vi "Configure Function Mode of Source.vi"(8 "error in":errorcluster, 10 "Mode":u16(ring) items=["Fixed", "List", "Battery", "Solar", "CarProfile", "Fuel", "Step"], 11 "VISA resource name":refnum<visa-resource-name>) -> (0 "error out":errorcluster, 3 "VISA resource name out":refnum<visa-resource-name>)   [LabVIEW 2015, in "IT-M3900C.lvlib"]
doc: "This command is used to set the power supply function mode.\n<b>Mode</b>\n0:Fixed\n1:List\n2:Battery\n3:Solar\n4:CarProfile\n5:Fuel\n6:Step"
uses:
  <instrlib>/IT-M3900C/IT-M3900C.lvlib
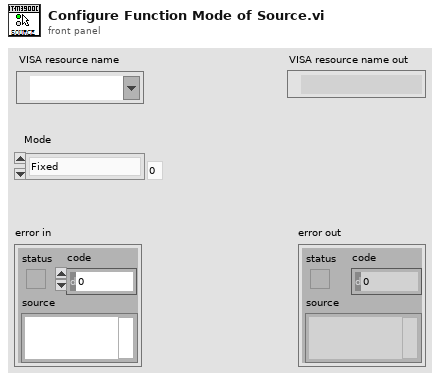
[diagram p1: front panel]
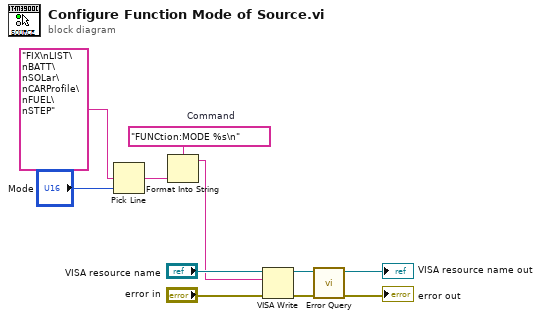
[diagram p0: block diagram]
diagram:
  w5 = "FUNCtion:MODE %s\n"  # Command
  n1 = Pick Line(multi-line string="FIX\nLIST\nBATT\nSOLar\nCARProfile\nFUEL\nSTEP", line index="Mode") -> (output string=w1:string)  [unwired: 1 in]
  n2 = Format Into String(format string=w5, w1) -> (resulting string=w4:string)  [unwired: 2 in, 1 out]
  n3 = VISA Write(VISA resource name="VISA resource name", write buffer=w4, error in (no error)="error in") -> (VISA resource name out=w8:refnum<visa-resource-name>, error out=w9:errorcluster)  [unwired: 1 out]
  n4 = call <instrlib>:"Error Query.vi"("error in"=w9, "VISA resource name"=w8) -> ("error out"=→"error out":errorcluster, "VISA resource name out"=→"VISA resource name out":refnum<visa-resource-name>)  [unwired: 6 in, 2 out]
